vi "Config Acquisition.vi"(0 "VISA resource name":refnum<visa-resource-name>, 5 "Record Length (0: 100000)":u16(ring) items=["100000", "1000000", "4000000", "R-Continuous"], 7 "Record Division (F: OFF)":bool, 9 "Time Base (F: Internal)":bool, 11 "error in (no error)":errorcluster) -> (4 "VISA resource name out":refnum<visa-resource-name>, 15 "error out":errorcluster)   [LabVIEW 2013, in "Yokogawa PZ4000.lvlib"]
doc: "This VI sends the Acquisition group command to the PZ4000 series.\nConfigure Control Functions are Record Length, Record Division, and Time Base."
uses:
  Yokogawa PZ4000.lvlib
panel:
  # "ON\nOFF"
  # "External\nInternal"
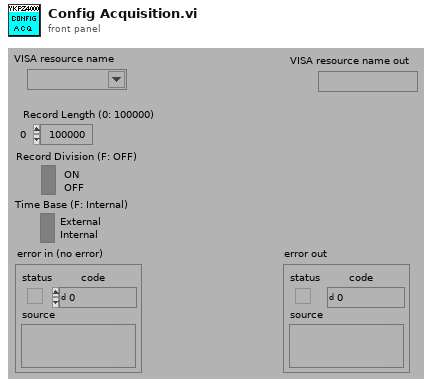
[diagram p1: front panel]
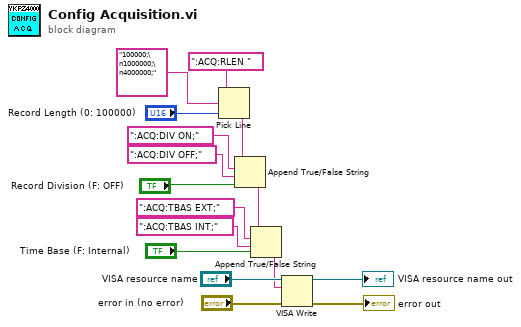
[diagram p0: block diagram]
diagram:
  n1 = Pick Line(string ("")=":ACQ:RLEN ", multi-line string="100000;\n1000000;\n4000000;", line index="Record Length (0: 100000)") -> (output string=w3:string)
  n2 = Append True/False String(1:"Record Division (F: OFF)", 2:":ACQ:DIV OFF;", 3:":ACQ:DIV ON;", 4:w3) -> (0:w2:string)
  n3 = Append True/False String(1:"Time Base (F: Internal)", 2:":ACQ:TBAS INT;", 3:":ACQ:TBAS EXT;", 4:w2) -> (0:w1:string)
  n4 = VISA Write(VISA resource name="VISA resource name", write buffer=w1, error in (no error)="error in (no error)") -> (VISA resource name out=→"VISA resource name out":refnum<visa-resource-name>, error out=→"error out":errorcluster)  [unwired: 1 out]
